vi "tool call.vi"(8 "error in":errorcluster, 10 "id in":i32, 11 "message json":string) -> (0 "error out":errorcluster, 3 "response":string)   [LabVIEW 2020, in "MCP Server.lvlib"]
uses:
  MCP Server.lvlib
  affbca46-cbce-409b-bfea-a62add01a465.vi
  <vilib>/JDP Science/JSONtext/Next JSON Value.vi
  <vilib>/JDP Science/JSONtext/String Subset.vi
  <vilib>/JDP Science/JSONtext/Parsing/Advance past next JSON Value (inlined COPY).vi
  <vilib>/JDP Science/JSONtext/Parsing/Advance past whitespace.vi
  <vilib>/JDP Science/JSONtext/Parsing/Advance past String.vi
  <vilib>/JDP Science/JSONtext/Parsing/Advance past Number.vi
  <vilib>/JDP Science/JSONtext/Parsing/Advance past Line Ending.vi
  <vilib>/JDP Science/JSONtext/Parsing/Parse Full Path or Item Name.vi
  <vilib>/JDP Science/JSONtext/Parsing/Advance past Array.vi
  <vilib>/JDP Science/JSONtext/Parsing/Advance past Object.vi
  <vilib>/JDP Science/JSONtext/support/Error Cluster From Code.vi
  <vilib>/JDP Science/JSONtext/Offset/Find Item Locations by Path.vi
  <vilib>/JDP Science/JSONtext/JSON text to Variant.vi
  <vilib>/JDP Science/JSONtext/LVClass Serializer/JSONtext LVClass Serializer.lvclass
  <vilib>/JDP Science/JSONtext/JSONtext.lvlib
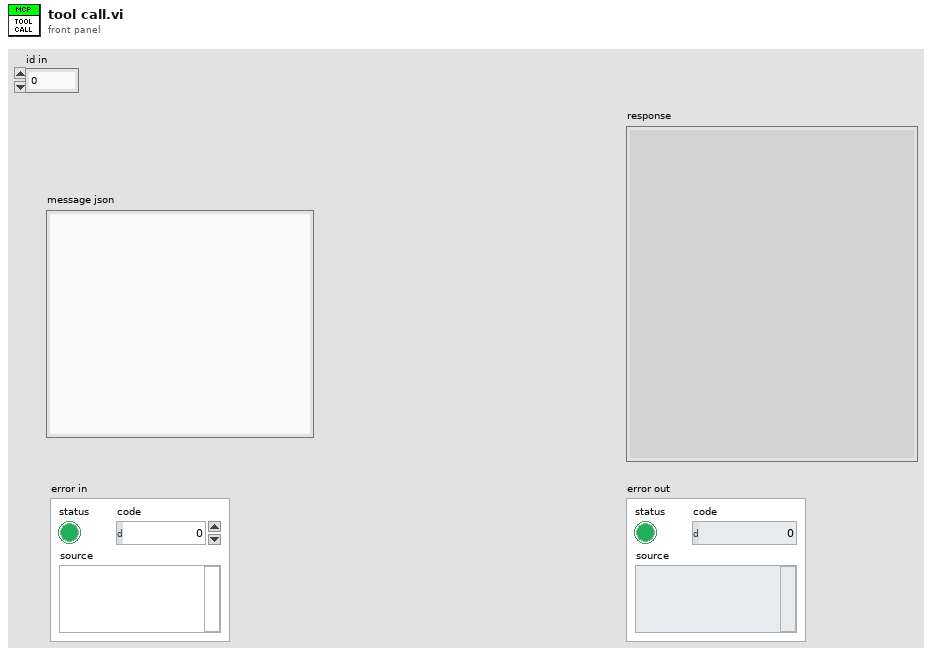
[diagram p1: front panel]
types:
  T1 = typedef "MCP Server.lvlib/Tool Data.ctl" = cluster{"Name":string, "Description":string, "Ignored":string[], "inputs":T2[], "outputs":T3[], "VI Refnum":refnum<vi>}
  T2 = typedef "MCP Server.lvlib/Input Parameter.ctl" = cluster{"name":string, "type":string, "description":string, "required":bool, "raw name":string}
  T3 = typedef "MCP Server.lvlib/Output Parameter.ctl" = cluster{"name":string, "description":string, "type":string, "raw name":string}
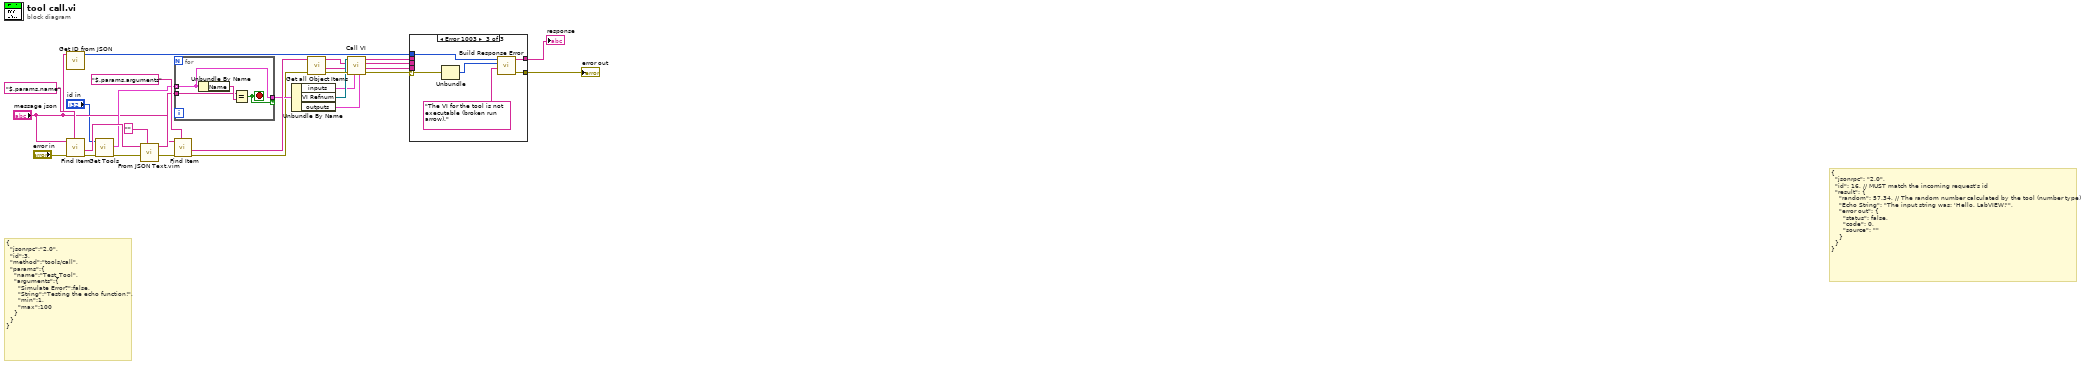
[diagram p0: block diagram]
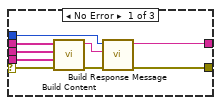
[diagram p2: hidden frame]
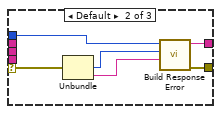
[diagram p3: hidden frame]
diagram:
  # "{\n  \"jsonrpc\": \"2.0\",\n  \"id\": 16, // MUST match the incoming request's id\n  \"result\": {\n    \"random\": 57.34, // The random number calculated by the tool (number type)\n    \"Echo String\": \"The input string was: 'Hello, LabVIEW!'\",\n    \"error out\": {\n      \"status\": false,\n      \"code\": 0,\n      \"source\": \"\"\n    }\n  }\n}"
  # "{\n  \"jsonrpc\":\"2.0\",\n  \"id\":3,\n  \"method\":\"tools/call\",\n  \"params\":{\n    \"name\":\"Test_Tool\",\n    \"arguments\":{\n      \"Simulate Error?\":false,\n      \"String\":\"Testing the echo function!\",\n      \"min\":1,\n      \"max\":100\n    }\n  }\n}"
  n1 = call "Get ID from JSON.vi"("message json"="message json") -> ("Data out"=w24:i32)  [unwired: 10 in]
  n2 = call <vilib>:"Find Item.vi"("$Path or Item Name"="$.params.name", "error in (no error)"="error in", "JSON"="message json") -> ("error out"=w11:errorcluster, "<JSON>"=w22:string)  [unwired: 5 in, 2 out]
  n3 = call "Get Tools.vi"("error in (no error)"=w11, "server id in"="id in") -> ("error out"=w12:errorcluster, "Tools"=w19:T1[])  [unwired: 7 in, 1 out]
  n4 = call "From JSON Text.vim"("Data Type and Default Value"="" ("$Path or Item Name"), "error in (no error)"=w12, "JSON"=w22) -> ("error out"=w10:errorcluster, "Data out"=w21:string)  [unwired: 7 in]
  n5 = for {
    tunnel: w19 -> [w30] mode=indexing
    tunnel: w21 -> [w31]
    tunnel: [w30] -> w18 if=w29
    stop <- w29 stop-if-true
    n6 = Unbundle By Name(w30) -> ("Name"=w32:string)
    n7 = Equal?(x=w31, y=w32) -> (x = y?=w29:bool)
  }
  n8 = call <vilib>:"Find Item.vi"("$Path or Item Name"="$.params.arguments", "error in (no error)"=w10, "JSON"="message json") -> ("error out"=w9:errorcluster, "<JSON>"=w27:string)  [unwired: 5 in, 2 out]
  n9 = Unbundle By Name(w18) -> ("inputs"=w3:T2[], "VI Refnum"=w6:refnum<vi>, "outputs"=w2:T3[])
  n10 = call <vilib>:"Get all Object Items.vi"("error in (no error)"=w9, "JSON"=w27) -> ("error out"=w8:errorcluster, "<JSON>"=w4:string[], "Item Names"=w5:string[])  [unwired: 6 in, 1 out]
  n11 = call "Call VI.vi"("output info"=w2, "input info"=w3, "error in (no error)"=w8, "Input Values"=w4, "Input Names"=w5, "VI in"=w6) -> ("error out"=w1:errorcluster, "output values"=w26:string[], "output names"=w25:string[], "pictures"=w15:string[])  [unwired: 2 in]
  n12 = case shown="Error 1003" w1 {
    selector: w1 -> [w33 w46 w52]
    tunnel: w26 -> [w41 _ _]
    tunnel: w25 -> [w40 _ _]
    tunnel: w24 -> [w39 w43 w50]
    tunnel: [w37 w42 w49] -> w17
    tunnel: w15 -> [w36 _ _]
    tunnel: [w35 w47 w53] -> w7
    frame No Error {
      n13 = call "Build Content.vi"("error in (no error)"=w33, "values"=w41, "names"=w40, "pictures"=w36) -> ("error out"=w34:errorcluster, "<JSON>"=w38:string)  [unwired: 6 in]
      n14 = call "Build Response Message.vi"("error in (no error)"=w34, "Result content"=w38, "message id in"=w39) -> ("error out"=w35:errorcluster, "MCP message out"=w37:string)  [unwired: 7 in]
    }
    frame Default {
      n15 = Unbundle(w46) -> ("code"=w45:i32, "source"=w44:string)  [unwired: 1 out]
      n16 = call "Build Response Error.vi"("message"=w44, "code"=w45, "message id in"=w43) -> ("error out"=w47:errorcluster, "MCP message out"=w42:string)  [unwired: 7 in]
    }
    frame Error {
      n17 = Unbundle(w52) -> ("code"=w51:i32)  [unwired: 2 out]
      n18 = call "Build Response Error.vi"("message"="The VI for the tool is not executable (broken run arrow).", "code"=w51, "message id in"=w50) -> ("error out"=w53:errorcluster, "MCP message out"=w49:string)  [unwired: 7 in]
    }
  }
  "error out" <- w7
  "response" <- w17
